vi "User Event-Minimize-Value Change.vi"(8 "Error In":errorcluster, 11 "Appearance Actor in":refnum<class "Appearance Actor.lvclass">) -> (0 "Error Out":errorcluster, 3 "Appearance Actor out":refnum<class "Appearance Actor.lvclass">)   [LabVIEW 2021, in "Appearance Actor.lvlib" / "Appearance Actor.lvclass"]
doc: "Handles Minimize Event. By Default, minimizes the FP Window if possible (else return an error). Override this method to change its behavior."
uses:
  Appearance Actor.lvclass
  Appearance Actor.lvclass/Appearance Actor.ctl
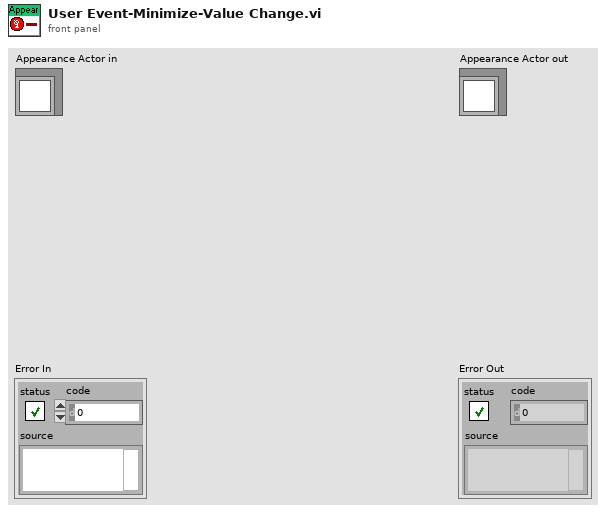
[diagram p1: front panel]
types:
  T1 = enum32{"Invalid", "Standard", "Closed", "Hidden", "Minimized", "Maximized"}
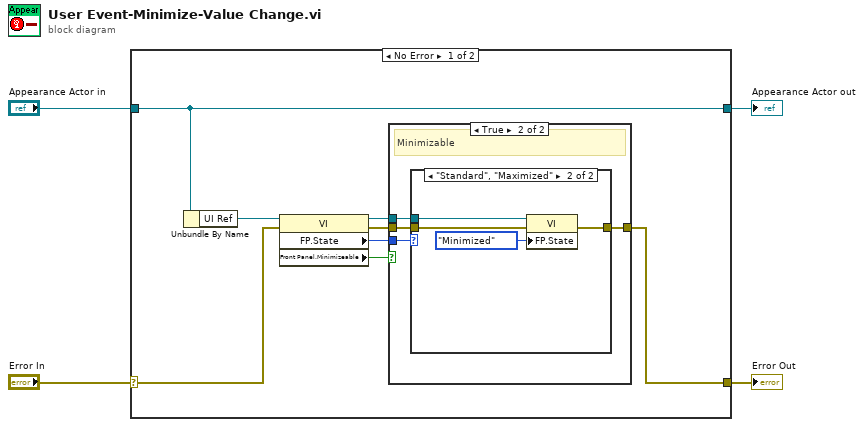
[diagram p0: block diagram]
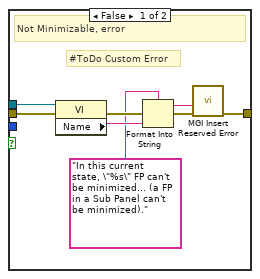
[diagram p2: hidden frame]
diagram:
  n1 = case shown="No Error" "Error In" {
    selector: "Error In" -> [w10 w31]
    tunnel: [w6 w31] -> w3
    tunnel: [w12 w30] -> w1
    tunnel: "Appearance Actor in" -> [w12 w30]
    frame No Error {
      n2 = Unbundle By Name(w12) -> ("UI Ref"=w11:refnum<vi>)
      n3 = property class="VI"(reference=w11, error in=w10) -> (reference out=w8:refnum<vi>, error out=w9:errorcluster, "FP.State"=w7:T1, "Front Panel.Minimizeable"=w5:bool)
      n4 = case shown="True" w5 {
        tunnel: w9 -> [w18 w24]
        tunnel: w8 -> [w19 w23]
        tunnel: w7 -> [_ w22]
        tunnel: [w20 w21] -> w6
        frame False {
          # "#ToDo Custom Error"
          # "Not Minimizable, error"
          n5 = property class="VI"(reference=w19, error in=w18) -> (error out=w15:errorcluster, "Name"=w14:string)  [unwired: 1 out]
          n6 = Format Into String(format string="In this current state, \"%s\" FP can't be minimized... (a FP in a Sub Panel can't be minimized)." ("Error Description"), error in=w15, w14) -> (resulting string=w17:string, error out=w16:errorcluster)  [unwired: 1 in]
          n7 = call <userlib>:"MGI Insert Reserved Error.vi"("Error In"=w16, "Error Description"=w17) -> ("Error Out"=w20:errorcluster)  [unwired: 9 in]
        }
        frame True {
          # "Minimizable"
          n8 = case shown="\"Standard\", \"Maximized\"" w22 {
            tunnel: w24 -> [w25 w28]
            tunnel: w23 -> [_ w29]
            tunnel: [w25 w26] -> w21
            frame Default {
              # "#ToDo Error?"
            }
            frame "Standard", "Maximized" {
              n9 = property class="VI"(reference=w29, error in=w28, "FP.State"=T1."Minimized" ("Front Panel Window:State")) -> (error out=w26:errorcluster)  [unwired: 1 out]
            }
          }
        }
      }
    }
    frame Error {
    }
  }
  "Error Out" <- w3
  "Appearance Actor out" <- w1
